vi "Color_AddSpaces.vi"(7 "Text.Selection":T1, 8 "Add Spaces?":bool, 11 "String in":refnum<vi>) -> (1 "Cursor":cluster{u32, u32}, 3 "String out":refnum<vi>)   [LabVIEW 2024]
uses:
  <vilib>/Utility/miscctls.llb/LVSelectionTypeDef.ctl
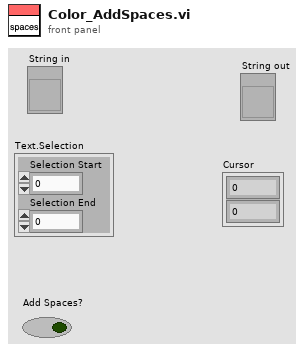
[diagram p1: front panel]
types:
  T1 = typedef "LVSelectionTypeDef.ctl" = cluster{"Selection Start":u32, "Selection End":u32}
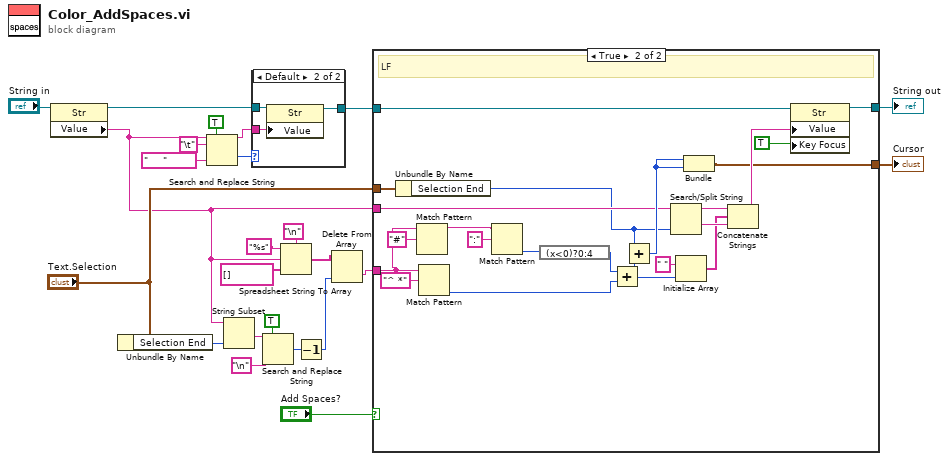
[diagram p0: block diagram]
diagram:
  n1 = property on="Property Node" class="Str"(reference="String in") -> (reference out=w6:refnum<vi>, "Value"=w5:string)  [unwired: 1 in, 1 out]
  n2 = Unbundle By Name("Text.Selection") -> ("Selection End"=w20:u32)
  n3 = Search and Replace String(replace all?=TRUE ("replace all? (F)"), input string=w5, search string="\t", replace string="     " ("replace string (\"\")")) -> (result string=w9:string, number of replacements=w10:i32)  [unwired: 4 in, 2 out]
  n4 = String Subset(string=w5, length (rest)=w20) -> (substring=w19:string)  [unwired: 1 in]
  n5 = case shown="Default" w10 {
    tunnel: w6 -> [w25 w28]
    tunnel: [w25 w27] -> w8
    tunnel: w9 -> [_ w26]
    frame 0 {
    }
    frame Default {
      n6 = property on="Property Node" class="Str"(reference=w28, "Value"=w26) -> (reference out=w27:refnum<vi>)  [unwired: 1 in, 1 out]
    }
  }
  n7 = Search and Replace String(replace all?=TRUE ("replace all? (F)"), input string=w19, search string="\n") -> (number of replacements=w16:i32)  [unwired: 5 in, 3 out]
  n8 = Spreadsheet String To Array(delimiter (Tab)="\n", format string="%s", spreadsheet string=w5, array type (2D Dbl)=string[] []) -> (array=w1:string[])
  n9 = Decrement(x=w16) -> (x-1=w15:i32)
  n10 = Delete From Array(array=w1, index=w15) -> (deleted portion=w24:string)  [unwired: 1 in, 1 out]
  n11 = case shown="True" "Add Spaces?" {
    tunnel: w24 -> [_ w51]
    tunnel: w5 -> [_ w38]
    tunnel: w8 -> [w29 w44]
    tunnel: [w29 w43] -> w23
    tunnel: "Text.Selection" -> [w30 w40]
    tunnel: [w30 w34] -> w14
    frame False {
    }
    frame True {
      # "LF"
      n12 = Unbundle By Name(w40) -> ("Selection End"=w37:u32)
      n13 = Match Pattern(string=w51, regular expression="#") -> (before substring=w48:string)  [unwired: 1 in, 3 out]
      n14 = Match Pattern(string=w51, regular expression="^ *") -> (offset past match=w45:i32)  [unwired: 1 in, 3 out]
      n15 = Match Pattern(string=w48, regular expression=":") -> (offset past match=w47:i32)  [unwired: 1 in, 3 out]
      n16 = expression code="(x<0)?0:4"(w47) -> (w46:i32)
      n17 = Add(x=w46, y=w45) -> (x+y=w33:i32)
      n18 = Add(x=w37, y=w33) -> (x+y=w39:u32)
      n19 = Search/Split String(string=w38, offset (0)=w37) -> (substring before match=w36:string, match + rest of string=w35:string)  [unwired: 1 in, 1 out]
      n20 = Initialize Array(" " ("regular expression"), w33) -> (w31:string[])
      n21 = Bundle(w39, w39) -> (w34:cluster{u32, u32})  [unwired: 1 in]
      n22 = Concatenate Strings(w36, w31, w35) -> (w42:string)
      n23 = property class="Str"(reference=w44, "Value"=w42, "Key Focus"=TRUE) -> (reference out=w43:refnum<vi>)  [unwired: 1 in, 1 out]
    }
  }
  "String out" <- w23
  "Cursor" <- w14
